vi "Write Constants to Robot.vi"(10 "Variable Names":string[](array[string]), 11 "Array of Numbers":dbl[](array[numeric])) -> ()   [LabVIEW 2013]
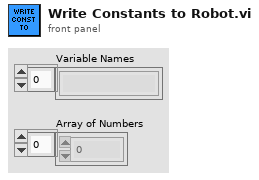
[diagram p1: front panel]
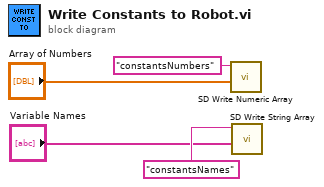
[diagram p0: block diagram]
diagram:
  n1 = call <vilib>:"SD Write Numeric Array.vi"("Numeric Array"="Array of Numbers", "Name"="constantsNumbers") -> ()  [unwired: 8 in, 2 out]
  n2 = call <vilib>:"SD Write String Array.vi"("String Array"="Variable Names", "Name"="constantsNames") -> ()  [unwired: 8 in, 2 out]
